vi "HW6.vi"() -> ()   [LabVIEW 2011]
panel:
  in  "Stop (F)":bool
  out "Vy":dbl
  out "Vx":dbl
  in  "I in":dbl
  out "Iout":dbl
  in  "speed":dbl
  in  "?":bool
  out "Array of points":cluster{"x":dbl, "x":dbl}[](array[cluster])
  out "Number of points":dbl
  out "new picture":picture
  out "Image Out":T1(plugin-control)
  in  "Color Box":u32(colorbox)=13816530
  # "This is an image processing base omni Robot path drawer.\nFor using @ first you need a red white board marker \nthen push the \"space\" for start drawing and push \"E\" for Stop.\nafter that you have robot speed in each point."
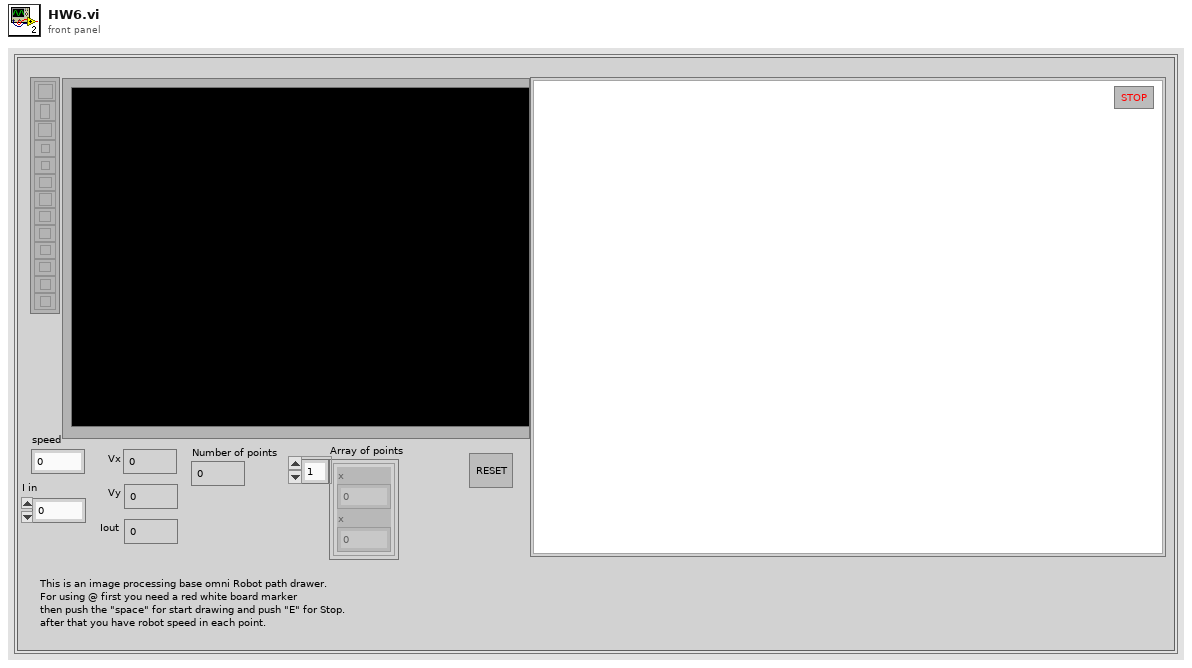
[diagram p1: front panel]
types:
  T1 = typedef "IMAQ Image.ctl" = refnum<image>
  T2 = cluster{"Width":u16, "Style":enum32{"Solid", "Dash", "Dot", "DashDot", "DashDotDot"}}
  T3 = cluster{"Position":cluster{"x":sgl, "y":sgl}, "Angle":sgl, "Scale":sgl, "Score":sgl, "Bounding Box":cluster{"x":sgl, "y":sgl}[]}[]
  T4 = cluster{"Calibrated Matches (Color Pattern Matching 1)[0]":cluster{"Position":cluster{"x":sgl, "y":sgl}, "Angle":sgl, "Scale":sgl, "Score":sgl, "Bounding Box":cluster{"x":sgl, "y":sgl}[]}, "Calibrated Matches (Color Pattern Matching 1)[1]":cluster{"Position":cluster{"x":sgl, "y":sgl}, "Angle":sgl, "Scale":sgl, "Score":sgl, "Bounding Box":cluster{"x":sgl, "y":sgl}[]}, "Calibrated Matches (Color Pattern Matching 1)[2]":cluster{"Position":cluster{"x":sgl, "y":sgl}, "Angle":sgl, "Scale":sgl, "Score":sgl, "Bounding Box":cluster{"x":sgl, "y":sgl}[]}, "Calibrated Matches (Color Pattern Matching 1)[3]":cluster{"Position":cluster{"x":sgl, "y":sgl}, "Angle":sgl, "Scale":sgl, "Score":sgl, "Bounding Box":cluster{"x":sgl, "y":sgl}[]}, "Calibrated Matches (Color Pattern Matching 1)[4]":cluster{"Position":cluster{"x":sgl, "y":sgl}, "Angle":sgl, "Scale":sgl, "Score":sgl, "Bounding Box":cluster{"x":sgl, "y":sgl}[]}, "Calibrated Matches (Color Pattern Matching 1)[5]":cluster{"Position":cluster{"x":sgl, "y":sgl}, "Angle":sgl, "Scale":sgl, "Score":sgl, "Bounding Box":cluster{"x":sgl, "y":sgl}[]}, "Calibrated Matches (Color Pattern Matching 1)[6]":cluster{"Position":cluster{"x":sgl, "y":sgl}, "Angle":sgl, "Scale":sgl, "Score":sgl, "Bounding Box":cluster{"x":sgl, "y":sgl}[]}, "Calibrated Matches (Color Pattern Matching 1)[7]":cluster{"Position":cluster{"x":sgl, "y":sgl}, "Angle":sgl, "Scale":sgl, "Score":sgl, "Bounding Box":cluster{"x":sgl, "y":sgl}[]}, "Calibrated Matches (Color Pattern Matching 1)[8]":cluster{"Position":cluster{"x":sgl, "y":sgl}, "Angle":sgl, "Scale":sgl, "Score":sgl, "Bounding Box":cluster{"x":sgl, "y":sgl}[]}}
  T5 = cluster{"Position":cluster{"x":sgl, "y":sgl}, "Angle":sgl, "Scale":sgl, "Score":sgl, "Bounding Box":cluster{"x":sgl, "y":sgl}[]}
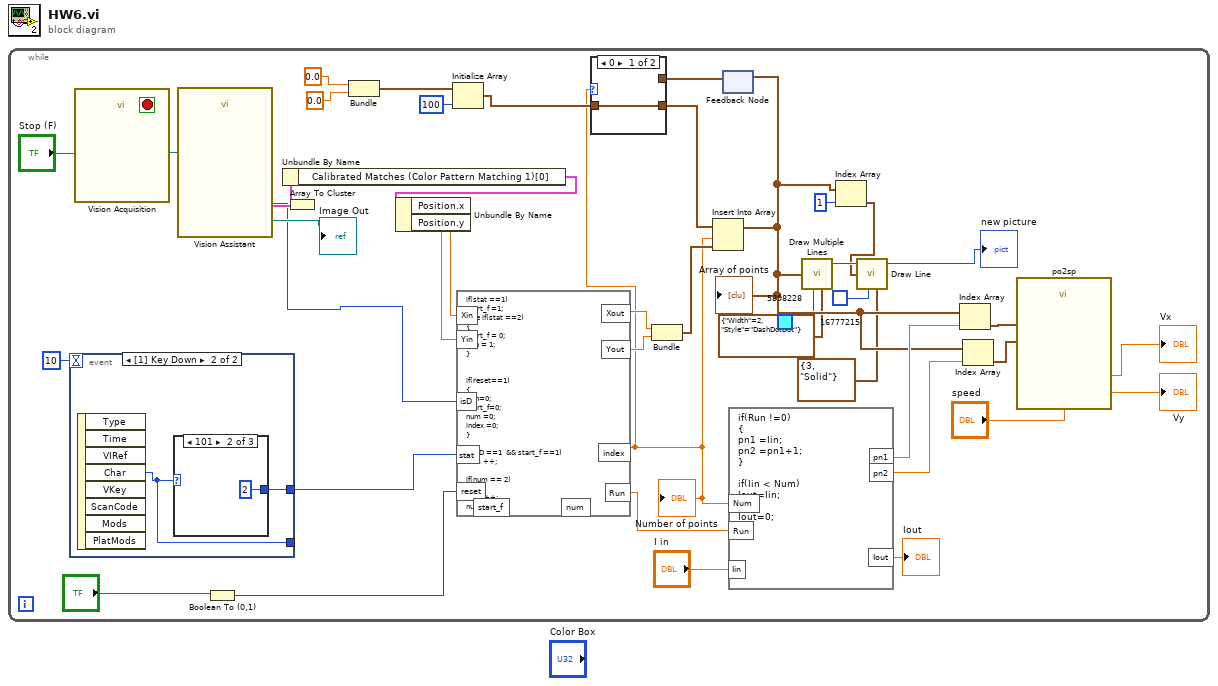
[diagram p0: block diagram]
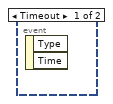
[diagram p2: hidden frame]
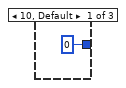
[diagram p3: hidden frame]
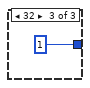
[diagram p4: hidden frame]
diagram:
  n1 = while {
    stop <- w43 stop-if-true
    n2 = event shown="[1] Key Down" {
      selector: _ -> [_ _]
      dyn-events: _ -> [_ _]
      timeout: 10 -> [_ _]
      tunnel: [_ w46] -> w21
      tunnel: [_ w45] -> _
      event Timeout {
        n3 = event-data() -> ()  [unwired: 1 in, 2 out]
      }
      event Key Down {
        n4 = event-data() -> ("Char"=w45:i16)  [unwired: 1 in, 7 out]
        n5 = case shown="101" w45 {
          tunnel: [0 2 1] -> w46
          frame 10, Default {
          }
          frame 101 {
          }
          frame 32 {
          }
        }
      }
    }
    n6 = call "Vision Acquisition"("Stop (F)"="Stop (F)") -> ("Image Out"=w42:T1, "Stopped"=w43:bool)  [unwired: 24 in, 1 out]
    n7 = call "Vision Assistant"("Image In"=w42) -> ("Image Out"=→"Image Out":T1, "Calibrated Matches (Color Pattern Matching 1)"=w41:T3, "Number of Matches (Color Pattern Matching 1)"=w39:i32)  [unwired: 23 in, 1 out]
    n8 = Boolean To (0,1)(Boolean="?") -> (0, 1=w30:i16)
    n9 = Array To Cluster(array=w41) -> (cluster=w29:T4)
    n10 = Unbundle By Name(w29) -> ("Calibrated Matches (Color Pattern Matching 1)[0]"=w28:T5)
    n11 = Bundle("x"=0.0, "x"=0.0) -> (w35:cluster{"x":dbl, "x":dbl})  [unwired: 1 in]
    n12 = Unbundle By Name(w28) -> ("Position.x"=w27:sgl, "Position.y"=w26:sgl)
    n13 = Initialize Array(w35, 100 ("dimension size")) -> (w34:cluster{"x":dbl, "x":dbl}[])
    n14 = formula code="if(stat ==1)\nstart_f =1;\nelse if(stat ==2)\n{\nstart_f = 0;\nRun = 1;\n}\n\n\nif(reset==1)\n{\nRun=0;\nstart_f=0;\nnum =0;\nindex =0;\n}\n\nif(isD ==1  && start_f ==1)\nnum ++;\n\nif(num == 2)\n{\nindex++;\nnum=0;\nXout = 640 - Xin;\nYout= Yin;\n}"("isD"=w39, "reset"=w30, "Xin"=w27, "Yin"=w26, "stat"=w21) -> ("index"=w10:dbl, "Xout"=w25:dbl, "Yout"=w24:dbl, "Run"=w20:dbl)  [unwired: 2 out]
    "Number of points" <- w10
    n15 = Bundle("Xout"=w25, "Yout"=w24) -> (w23:cluster{"Xout":dbl, "Yout":dbl})  [unwired: 1 in]
    n16 = feedback #1() -> (w32:cluster{"x":dbl, "x":dbl}[])  [unwired: 1 in]
    n17 = case shown="0" w10 {
      tunnel: w34 -> [w50 _]
      tunnel: [w50 w51] -> w33
      tunnel: w32 -> [_ w51]
      frame 0 {
      }
      frame 1, Default {
      }
    }
    n18 = Insert Into Array(array=w33, index=w10, new element=w23) -> (w6:cluster{"x":dbl, "x":dbl}[])
    "Array of points" <- w6
    n19 = feedback-in #1(w6) -> ()
    n20 = formula code="if(Run !=0)\n{\npn1 =Iin;\npn2 =pn1+1;\n}\n\nif(Iin < Num)\nIout=Iin;\nelse\nIout=0;"("Run"=w20, "Num"=w10, "Iin"="I in") -> ("Iout"=→"Iout":dbl, "pn1"=w18:dbl, "pn2"=w19:dbl)
    n21 = call <vilib>:"Draw Multiple Lines.vi"("line endpoints"=w6, "color(black)"=u32 5898228, "pen"=T2 {"Width"=2, "Style"=enum."DashDotDot"}) -> ("new picture"=w9:picture)  [unwired: 6 in]
    n22 = Index Array(array=w6, index=1) -> (element=w5:cluster{"x":dbl, "x":dbl})
    n23 = call <vilib>:"Draw Line.vi"("picture"=w9, "end point"=w5, "color(black)"=u32 16777215, "pen"=T2 {"Width"=3, "Style"=enum."Solid"}) -> ("new picture"=→"new picture":picture)  [unwired: 5 in]
    n24 = Index Array(array=w6, index=w18) -> (element=w17:cluster{"x":dbl, "x":dbl})
    n25 = Index Array(array=w6, index=w19) -> (element=w16:cluster{"x":dbl, "x":dbl})
    n26 = call "po2sp.vi"("speed"="speed", "P2"=w16, "P1"=w17) -> ("Vx"=→"Vx":dbl, "Vy"=→"Vy":dbl)  [unwired: 7 in]
  }
